vi "Unsupported Type Error.vi"(8 "error in (no error)":errorcluster, 11 "Variant":variant) -> (0 "Unsupported Parameter Variant Type":errorcluster)   [LabVIEW 2020, in "RxnRover.lvlib"]
doc: "Provides an error cluster for an unsupported type. This will get the type of the variant and add that to the error message."
uses:
  RxnRover.lvlib
  <vilib>/Utility/Data Type/NI_Data Type.lvlib
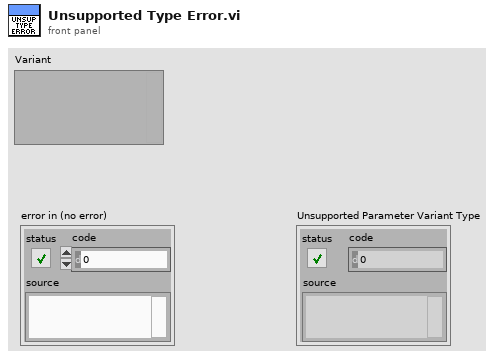
[diagram p1: front panel]
types:
  T1 = typedef "NI_Data Type.lvlib/Data Type.ctl" = enum8{"Invalid Type", "Void", "I8", "I16", "I32", "I64", "U8", "U16", "U32", "U64", "Single Float", "Double Float", "Extended Float", "Single Complex", "Double Complex", "Extended Complex", "Enum U8", "Enum U16", "Enum U32", "Enum U64", "Single Float With Unit", "Double Float With Unit", "Extended Float With Unit", "Single Complex with Unit", "Double Complex with Unit", "Extended Complex with Unit", "Boolean", "String", "Path", "Picture", "Tag", "Array", "Cluster", "Variant", "LV Variant", "Waveform", "Timestamp", "Digital Waveform", "Digital Data", "ExpressData", "Refnum", "External Data", "VI", "Poly VI", "LabVIEW Class Instance", "Fixed Point", "Set Collection", "Map Collection"}
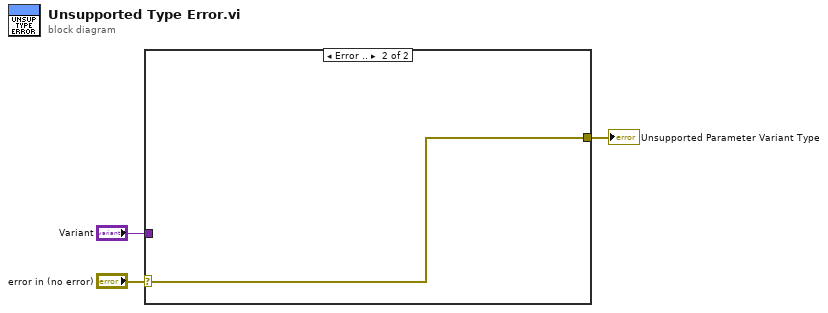
[diagram p0: block diagram]
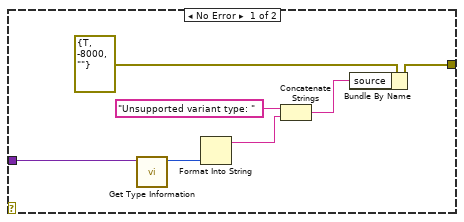
[diagram p2: hidden frame]
diagram:
  n1 = case shown="Error .." "error in (no error)" {
    selector: "error in (no error)" -> [_ w11]
    tunnel: [w8 w11] -> w3
    tunnel: "Variant" -> [w6 _]
    frame No Error {
      n2 = call <vilib>:"Get Type Information.vi"("variant"=w6) -> ("type"=w5:T1)  [unwired: 6 in, 4 out]
      n3 = Format Into String(w5) -> (resulting string=w4:string)  [unwired: 3 in, 1 out]
      n4 = Concatenate Strings("Unsupported variant type: " ("string"), w4) -> (w7:string)
      n5 = Bundle By Name(cluster=errorcluster {"status"=TRUE, "code"=-8000, "source"=""} ("Unsupported Parameter Variant Type"), "source"=w7) -> (w8:errorcluster)
    }
    frame Error {
    }
  }
  "Unsupported Parameter Variant Type" <- w3
